vi "UHR-Fleezers Control (host) -Leonardo 04-2018 V2.vi"(0 "Tab Control":T5(tab)=enum."Trap Control (RF)") -> ()   [LabVIEW 2013] (continued)
  n83 = local write "Ave. Period (s)"(w194) -> ()
  n84 = property on="2D or 1D Scan" class="Bool (strict)"("Val(Sgnl)"=w149) -> ()  [unwired: 2 in, 2 out]
  n85 = xnode "Read/Write Control"("FPGA VI Reference In"=w146, "error in"=w165, "ai count"="AI Count (ticks)", "Interlace ON/OFF"=w132, "Number Interlace Cycles"=w131, "Set 1"=w12, "Set 2"=w11, "Set 3"=w10, "FB On/Off Set 1"=w252, "FB On/Off Set 2"=w251, "Interlace Off Parameters"=w130, "FB Setpoint Set 1"=w243, "FB Setpoint Set 2"=w242, "FB Gains"="PID gains", "FB output range"=cluster{"output high":i16, "output low":i16} {"output high"=3000, "output low"=0} ("FB output range 1"), "Cycles per step"=w228, "Scan BD"=w240, "Number of scans"=w224, "Scan steps"=w229, "Scan freq.  increment"=w230, "AO1 (Y)"=w212, "AO2 (X)"=w211, "Scan freq.  increment (MCL)"=w205, "Scan steps (MCL)"=w204, "Cycles per step (MCL)"=w203, "Number of scans (MCL)"=w202, "MCL count"=w129, "Cont. Scan (MCL)"=w201, "MCL Scan Axis"=w195, "1D or 2D Scan?"=w149, "N of AI1 Int Acq Sets"=w185, "BD 1 Delay (ticks)"="Freq switch delay", "Amp switch delay"="Amp switch delay", "Swap F1 and F2"="Swap F1 and F2", "APD Acq Rate Count"=w154, "APD to FIFO"=FALSE, "APD Gate Operating Mode"="APD Gate", "APD Gate ON Count"="APD Gate ON Count", "APD Gate OFF Count"="APD Gate OFF Count", "Invert APD Gate"="Invert APD Gate", "DIO count 1 (ticks)"="DIO count 1 (ticks)", "DIO count 2 (ticks)"="DIO count 2 (ticks)", "DIO count 3 (ticks)"="DIO count 3 (ticks)", "APD 1 AO scale factor"="APD 1 AO Mult.", "APD 2 AO scale factor"="APD 2 AO Mult.", "Diff FB Measurement?"=w17, "Dynamic Force FB (Ronen)"=w16, "Negate Diff?"=w15, "Next trap write delay (ticks)"="Next trap write delay (ticks)", "Phase offset method"="Phase offset method", "Phase Trap 1"="Phase increment trap 1", "RF phase reset before cycles"="RF phase reset before cycles", "Phase Trap 2"="Phase increment trap 2") -> ("FPGA VI Reference Out"=w124:T20, "error out"=w126:errorcluster)  [unwired: 1 in]
  n86 = local read "Green Laser ON/Interlacing"() -> (w127:bool)
  n87 = local read "Green laser mode"() -> (w128:enum32{"Laser ON", "Laser OFF", "Interlace"})
  n88 = local read "GI Frequency, OFF count"() -> (w120:u32)
  n89 = local read "GI Frequency, ON count"() -> (w119:u32)
  n90 = Multiply(x="Current When FB OFF (%)", y=655.35) -> (x*y=w110:dbl)
  n91 = local read "Green FB Count"() -> (w118:u32)
  n92 = Multiply(x="Green FB Setpoint (mV)", y=3.2767) -> (x*y=w107:dbl)
  n93 = To Unsigned Word Integer(number=w110) -> (unsigned 16bit integer=w108:u16)
  n94 = local read "Invert GI"() -> (w122:bool)
  n95 = To Word Integer(number=w107) -> (16bit integer=w105:i16)
  n96 = case shown="True" w127 {
    tunnel: w128 -> [_ w287]
    tunnel: [enum32{"Laser ON", "Laser OFF", "Interlace"}."Laser OFF" ("Green laser mode") w287] -> w121
    frame False {
    }
    frame True {
    }
  }
  n97 = local read "Trap Pos. AI1 X Pre-scale"() -> (w78:u16)
  n98 = local read "Trap Pos FB Monitor\nT1 or T2"() -> (w85:bool)
  n99 = local read "Trap Pos FB Int Count"() -> (w73:u16)
  n100 = local read "Trap Pos FB Negate Action"() -> (w84:bool)
  n101 = local read "Trap Pos. FB Offset Factor"() -> (w83:i64)
  n102 = local read "Trap Pos. FB Mult Factor"() -> (w82:i64)
  n103 = local read "Trap Pos. FB Gains"() -> (w80:T11)
  n104 = local read "Trap Pos. FB Range"() -> (w81:T12)
  n105 = xnode "Read/Write Control"("FPGA VI Reference In"=w124, "error in"=w126, "Green interlace ON count 2"=w119, "Green interlace OFF count 2"=w120, "Invert GI 2"=w122, "Operating Mode 2"=w121, "Green FB Gains"="Green FB Gains", "Green FB Setpoint"=w105, "Green FB On/Off"="Green FB On/Off", "Current Out"=w108, "Green int current ON count adj"="Green int current ON count adj", "Green FB Count"=w118, "Operating Mode"=w121, "Green interlace OFF count"=w120, "Green interlace ON count"=w119, "Invert GI"=w122, "Trap Pos FB Monitor T1 or T2"=w85, "Trap Pos FB Negate Action"=w84, "Trap Pos. FB Offset Factor"=w83, "Trap Pos. FB Mult Factor"=w82, "Trap pos. FB Range"=w81, "Trap Pos. FB Gains"=w80, "Force feedback"=FALSE, "AI1 X Scale"=w78, "Trap Pos to FIFO"=TRUE, "Trap Pos FB Int Count"=w73) -> ("FPGA VI Reference Out"=w123:T20, "error out"=w125:errorcluster)
  n106 = xnode "Invoke Method"("FPGA VI Reference In"=w123, "error in"=w125, "Requested Depth"="Trap AI FIFO Depth") -> ("FPGA VI Reference Out"=w88:T20, "error out"=w87:errorcluster)  [unwired: 1 out]
  n107 = xnode "Invoke Method"("FPGA VI Reference In"=w88, "error in"=w87, "Requested Depth"="Trap Position FIFO Depth") -> ("FPGA VI Reference Out"=w75:T20, "error out"=w74:errorcluster)  [unwired: 1 out]
  n108 = flat-sequence {
    tunnel: w147 -> [w292]
    tunnel: [w292] -> w146
    tunnel: [w291] -> w33
    tunnel: [w290] -> w145
    tunnel: [w288] -> w143
    tunnel: [w289] -> w144
    frame #0 {
      w289 = T16 {"Minimum"=60.0, "Maximum"=90.0, "Increment"=1.0} ("Min Max Inc")
      w288 = T16 {"Minimum"=0.0, "Maximum"=75.0, "Increment"=1.0} ("Data Entry Limits")
      w291 = T16 {"Minimum"=60.0, "Maximum"=90.0, "Increment"=1.0} ("Min Max Inc")
      w290 = T16 {"Minimum"=0.0, "Maximum"=75.0, "Increment"=1.0} ("Data Entry Limits")
      n109 = property on="BD 2 Frequency 1 (MHz)" class="DigNum (strict)"("Data Range"=w289) -> ()  [unwired: 2 in, 2 out]
      n110 = property on="BD 2 Frequency 3 (MHz)" class="DigNum (strict)"("Data Range"=w289) -> ()  [unwired: 2 in, 2 out]
      n111 = property on="BD 2 Frequency 2 (MHz)" class="DigNum (strict)"("Data Range"=w289) -> ()  [unwired: 2 in, 2 out]
      n112 = property on="BD 1 Frequency 1 (MHz)" class="DigNum (strict)"("Data Range"=w291) -> ()  [unwired: 2 in, 2 out]
      n113 = property on="BD 1 Frequency 2 (MHz)" class="DigNum (strict)"("Data Range"=w291) -> ()  [unwired: 2 in, 2 out]
      n114 = property on="BD 1 Frequency 3 (MHz)" class="DigNum (strict)"("Data Range"=w291) -> ()  [unwired: 2 in, 2 out]
      n115 = property on="BD 2 Amplitude 1 (%)" class="DigNum (strict)"("Data Range"=w288) -> ()  [unwired: 2 in, 2 out]
      n116 = property on="BD 2 Amplitude 2 (%)" class="DigNum (strict)"("Data Range"=w288) -> ()  [unwired: 2 in, 2 out]
      n117 = property on="BD 2 Amplitude 3 (%)" class="DigNum (strict)"("Data Range"=w288) -> ()  [unwired: 2 in, 2 out]
      n118 = property on="BD 1 Amplitude 3 (%)" class="DigNum (strict)"("Data Range"=w290) -> ()  [unwired: 2 in, 2 out]
      n119 = property on="BD 1 Amplitude 2 (%)" class="DigNum (strict)"("Data Range"=w290) -> ()  [unwired: 2 in, 2 out]
      n120 = property on="BD 1 Amplitude 1 (%)" class="DigNum (strict)"("Data Range"=w290) -> ()  [unwired: 2 in, 2 out]
      "X RF Frequency Limits (MHz)" <- w291
      "X RF Amplitude Limits (%)" <- w290
      "Y RF Amplitude Limits (%)" <- w288
      "Y RF Frequency Limits (MHz)" <- w289
    }
  }
  n121 = xnode "Invoke Method"("FPGA VI Reference In"=w75, "error in"=w74) -> ("FPGA VI Reference Out"=w53:T20, "error out"=w52:errorcluster)  [unwired: 1 in]
  n122 = flat-sequence "Initial FPGA Loop Relative Phase Adjustment" {
    tunnel: "Initial Phase Adjustment (GI) 2" -> [w294]
    tunnel: "Initial Phase Adj. (MCL)" -> [w295]
    tunnel: w52 -> [w296]
    tunnel: w53 -> [w297]
    tunnel: "Initial Phase Adjustment (GI)" -> [w298]
    tunnel: "Initial Phase Adjustment (AI1)" -> [w299]
    tunnel: [w299] -> w61
    tunnel: [w298] -> w60
    tunnel: [w297] -> w59
    tunnel: [w296] -> w58
    tunnel: [w295] -> w57
    tunnel: [w294] -> w56
    tunnel: [w310] -> w171
    tunnel: [w304] -> w169
    tunnel: "Initial Phase Adjustment (APD Acq)" -> [w303]
    tunnel: "Initial Phase Adjustment (APD 1 Gate)" -> [w302]
    tunnel: "Initial Phase Adjustment (Green FB)" -> [w301]
    tunnel: w61 -> [w309]
    tunnel: w60 -> [w308]
    tunnel: w59 -> [w307]
    tunnel: w58 -> [w306]
    tunnel: w57 -> [w305]
    tunnel: w56 -> [w300]
    tunnel: w171 -> [w312]
    tunnel: [w313] -> w170
    tunnel: w169 -> [w313]
    tunnel: [w312] -> w168
    tunnel: w170 -> [w316]
    tunnel: w168 -> [w315]
    tunnel: [w318] -> w167
    tunnel: [w317] -> w166
    tunnel: [w320] -> w51
    tunnel: [w321] -> w54
    tunnel: w167 -> [w321]
    tunnel: w166 -> [w320]
    frame #0 {
      n123 = Wait (ms)(milliseconds to wait=u32 1000) -> ()  [unwired: 1 out]
    }
    frame #1 {
      n124 = xnode "Read/Write Control"("FPGA VI Reference In"=w307, "error in"=w306, "Phase count adjustment"=w309, "Phase count adjustment (GI)"=w308, "Phase count adjustment (MCL)"=w305, "Phase Count Adjustment (APD Acq)"=w303, "Phase count adjustment (APD 1 Gate)"=w302, "Phase count adjustment (Green FB)"=w301, "Phase count adjustment (GI) 2"=w300) -> ("FPGA VI Reference Out"=w304:T20, "error out"=w310:errorcluster)
    }
    frame #2 {
      n125 = Wait (ms)(milliseconds to wait=u32 1000) -> ()  [unwired: 1 out]
    }
    frame #3 {
      w314 = TRUE
      n126 = xnode "Read/Write Control"("FPGA VI Reference In"=w316, "error in"=w315, "+ phase"=w314, "+ phase (GI)"=w314, "+ phase (MCL)"=w314, "+ phase (APD Acq)"=w314, "+ phase (APD 1 Gate)"=w314, "+ phase (Green FB)"=w314, "+ phase (GI) 2"=w314) -> ("FPGA VI Reference Out"=w317:T20, "error out"=w318:errorcluster)
    }
    frame #4 {
      n127 = Wait (ms)(milliseconds to wait=u32 1000) -> ()  [unwired: 1 out]
    }
  }
  n128 = Unbundle By Name(w33) -> ("Minimum"=w32:dbl, "Maximum"=w31:dbl)
  n129 = local read "Phase adj. (Green FB)"() -> (w141:i16)
  n130 = local read "Phase adj. (GI) 2"() -> (w111:i16)
  n131 = local read "Phase adjust (MCL)"() -> (w196:i16)
  n132 = local read "Phase adj. (AI1)"() -> (w198:i16)
  n133 = local read "Phase adj. (GI)"() -> (w197:i16)
  n134 = Multiply(x=w32, y=w30) -> (x*y=w28:dbl)
  n135 = Multiply(x=w31, y=w30) -> (x*y=w29:dbl)
  n136 = Multiply(x=49152000.0, y=6.0) -> (x*y=w22:dbl)
  n137 = Scale By Power Of 2(n=w27, x=w28) -> (x*2^n=w24:dbl)
  n138 = Scale By Power Of 2(n=w27, x=w29) -> (x*2^n=w23:dbl)
  n139 = xnode "Read/Write Control"("FPGA VI Reference In"=w51, "error in"=w54, "Phase count adjustment"=w198, "Phase count adjustment (GI)"=w197, "Phase count adjustment (MCL)"=w196, "Phase Count Adjustment (APD Acq)"="Phase Adj. (APD Acq)", "Phase count adjustment (APD 1 Gate)"="Phase Adj. (APD 1 Gate)", "Phase count adjustment (Green FB)"=w141, "Phase count adjustment (GI) 2"=w111) -> ("FPGA VI Reference Out"=w8:T20, "error out"=w7:errorcluster)
  n140 = Divide(x=w23, y=w22) -> (x/y=w20:dbl)
  n141 = Divide(x=w24, y=w22) -> (x/y=w21:dbl)
  n142 = To Unsigned Quad Integer(1:w21) -> (0:w19:u64)
  n143 = To Unsigned Quad Integer(1:w20) -> (0:w18:u64)
  n144 = xnode "Read/Write Control"("FPGA VI Reference In"=w8, "FB Min frequency"=w19, "FB Max Frequency"=w18) -> ()  [unwired: 1 in, 2 out]
  n145 = call "set RF board frequency - interlace.vi"("Board 2 Frequency Limits"=w144, "Board 1 Frequency Limits"=w33, "error in"=w7, "FPGA VI Reference In"=w8, "Board 2 Frequency 3 (MHz)"="BD 2 Frequency 3 (MHz)", "Board 1 Frequency 3 (MHz)"="BD 1 Frequency 3 (MHz)", "Board 2 Frequency 2 (MHz)"="BD 2 Frequency 2 (MHz)", "Board 2 Frequency 1 (MHz)"="BD 2 Frequency 1 (MHz)", "Board 1 Frequency 2 (MHz)"="BD 1 Frequency 2 (MHz)", "Board 1 Frequency 1  (MHz)"="BD 1 Frequency 1 (MHz)") -> ("error out"=w263:errorcluster, "FPGA VI Reference Out"=w264:T20)
  n146 = call "set RF board amplitude - interlace.vi"("Board 2 Amplitude Limits"=w143, "Board 1 Amplitude Limits"=w145, "error in"=w263, "FPGA VI Reference In"=w264, "Board 2 Amplitude 3 (%)"="BD 2 Amplitude 3 (%)", "Board 1 Amplitude 3 (%)"="BD 1 Amplitude 3 (%)", "Board 2 Amplitude 2 (%)"="BD 2 Amplitude 2 (%)", "Board 2 Amplitude 1 (%)"="BD 2 Amplitude 1 (%)", "Board 1 Amplitude 2 (%)"="BD 1 Amplitude 2 (%)", "Board 1 Amplitude 1 (%)"="BD 1 Amplitude 1 (%)") -> ("error out"=w49:errorcluster, "FPGA VI Reference Out"=w50:T20)
  n147 = flat-sequence {
    tunnel: w50 -> [w323]
    tunnel: w49 -> [w322]
    tunnel: [w323] -> w256
    tunnel: [w322] -> w255
    tunnel: [w331] -> w254
    tunnel: w256 -> [w331]
    tunnel: [w330] -> w253
    tunnel: w255 -> [w330]
    tunnel: w254 -> [w334]
    tunnel: w253 -> [w333]
    tunnel: [w334] -> w45
    tunnel: [w333] -> w44
    tunnel: [w340] -> w70
    tunnel: [w344] -> w55
    tunnel: w45 -> [w344]
    tunnel: w44 -> [w339]
    frame #0 {
      n148 = local read "Trap 1 (ON/OFF)"() -> (w324:bool)
      n149 = local write "Saving..."(FALSE ("Saving Data")) -> ()
      n150 = local write "Stop All"(FALSE ("Stop All")) -> ()
      n151 = local write "Index"(1.0 ("Index")) -> ()
      n152 = property on="Trap 1 ON" class="Bool (strict)"("Value"=w324) -> ()  [unwired: 2 in, 2 out]
      "Manipulating Trap" <- FALSE ("Manipulating Trap")
    }
    frame #1 {
      n153 = local read "Trap 2 (ON/OFF)"() -> (w329:bool)
      n154 = Wait (ms)(milliseconds to wait=u32 50) -> ()  [unwired: 1 out]
      n155 = property on="Trap 2 ON" class="Bool (strict)"("Val(Sgnl)"=w329) -> ()  [unwired: 2 in, 2 out]
    }
    frame #2 {
      n156 = local read "Scan Range (nm)"() -> (w335:dbl)
      n157 = call "Update messages.vi"("Message to add"="UHR-Fleezers ready.", "Old message string"="") -> ("New message string"=w338:string)
      n158 = local write "Messages"(w338) -> ()
      n159 = property on="Scan Range (nm)" class="DigNum (strict)"("Val(Sgnl)"=w335) -> ()  [unwired: 2 in, 2 out]
    }
    frame #3 {
      n160 = call "hamilton_controller.vi"("error in"=w339, "action"=T21."CONNECT") -> ("error out"=w341:errorcluster)  [unwired: 9 in]
      n161 = call "hamilton_controller.vi"("error in"=w341, "action"=T21."INITIALIZE VALVES") -> ("error out"=w340:errorcluster)  [unwired: 9 in]
    }
  }
  n162 = Subtract(x="BD 1 Frequency 1 (MHz)", y="BD 1 Frequency 2 (MHz)") -> (x-y=w184:dbl)
  n163 = Subtract(x="BD 2 Frequency 1 (MHz)", y="BD 2 Frequency 2 (MHz)") -> (x-y=w183:dbl)
  n164 = Square(x=w183) -> (x^2=w181:dbl)
  n165 = Square(x=w184) -> (x^2=w182:dbl)
  n166 = Add(x=w182, y=w181) -> (x+y=w180:dbl)
  n167 = Square Root(x=w180) -> (sqrt(x)=w179:dbl)
  n168 = local write "Trap Delta (MHz)"(w179) -> ()
  n169 = call "IMAQ Create"("Image Name"="APD 1 Image", "Image Type"=w94) -> ("New Image"=w93:T3)  [unwired: 3 in, 1 out]
  n170 = call "IMAQ Create"("Image Name"="APD 2 Image", "Image Type"=w94) -> ("New Image"=w92:T3)  [unwired: 3 in, 1 out]
  n171 = call "IMAQ Create"("Image Name"="Det. X Image", "Image Type"=w94) -> ("New Image"=w91:T3)  [unwired: 3 in, 1 out]
  n172 = call "IMAQ Create"("Image Name"="Det. Y Image", "Image Type"=w94) -> ("New Image"=w90:T3)  [unwired: 3 in, 1 out]
  n173 = Bundle("New Image"=w93, "New Image"=w92, "New Image"=w91, "New Image"=w90) -> (w89:T22)  [unwired: 1 in]
  n174 = Current VI's Path() -> (path=w34:path)
  n175 = Concatenate Strings("N.D.", "\r\n") -> (w38:string)
  n176 = Strip Path(path=w34) -> (stripped path=w35:path)  [unwired: 1 out]
  n177 = Initialize Array(w38, 4, 3) -> (w41:string[][])
  n178 = Build Path(base path=w35, name or relative path="Locations.txt") -> (appended path=→"Location path":path)
  n179 = local write "Location Matrix"(w41) -> ()
  n180 = while {
    stop <- w345 stop-if-true
    n181 = event shown="[0] Timeout" {
      selector: _ -> [_ _ _ _ _ _ _ _]
      dyn-events: _ -> [_ _ _ _ _ _ _ _]
      timeout: 10 -> [_ _ _ _ _ _ _ _]
      tunnel: [FALSE _ _ _ _ _ _ TRUE] -> w345
      event Timeout {
        # "Change the trajectory mode to Jog"
        # "Query and display stage positions"
        # "Setting ESP300 left and right limits for Z-axis, input in mm"
        # "Display Selected Location"
        n182 = event-data() -> ()  [unwired: 1 in, 2 out]
        n183 = local read "Capture Locations"() -> (w370:i32)
        n184 = local read "Location Matrix"() -> (w371:string[][])
        n185 = Concatenate Strings("1TP;\n2TP;\n3TP;\n1MD?;\n2MD?;\n3MD?" ("Substring"), "\r") -> (w354:string)
        n186 = local read "ESP Port"() -> (w357:refnum<visa-resource-name>)
        n187 = Index Array(array=w371, index (row)=w370) -> (element=w369:string[])  [unwired: 1 in]
        n188 = local read "ESP Port"() -> (w366:refnum<visa-resource-name>)
        n189 = VISA Write(VISA resource name=w357, write buffer=w354, error in (no error)="error in") -> (VISA resource name out=w355:refnum<visa-resource-name>, error out=w353:errorcluster)  [unwired: 1 out]
        n190 = Concatenate Strings("3SL" ("Substring"), "ESP ZL-Limit", ";3SR", "ESP ZR-Limit", "\r") -> (w365:string)
        n191 = Array To Cluster(array=w369) -> (cluster=w368:T23)
        n192 = case shown="True" TRUE ("Case Constant\n(See Context Help)") {
          tunnel: w355 -> [_ w409]
          tunnel: w353 -> [w390 w408]
          tunnel: [w390 w392] -> w359
          frame False {
          }
          frame True {
            w402 = u16 10 items=["1.0"=10, "1.5"=15, "2.0"=20] ("Serial Settings:Stop Bits")
            w403 = u16 0 items=["None", "Odd", "Even", "Mark", "Space"] ("Serial Settings:Parity")
            n193 = property class="Instr"(reference=w409, error in=w408, "Baud"=u32 921600 ("Serial Settings:Baud Rate"), "Data Bits"=u16 8 ("Serial Settings:Data Bits"), "Parity"=w403, "Stop Bits"=w402) -> (reference out=w407:refnum<visa-resource-name>, error out=w406:errorcluster, "Bytes at Port"=w391:u32)
            n194 = Wait (ms)(milliseconds to wait=u32 10) -> ()  [unwired: 1 out]
            n195 = VISA Read(VISA resource name=w407, byte count=w391, error in (no error)=w406) -> (VISA resource name out=w415:refnum<visa-resource-name>, read buffer=→"X Pos":string, error out=w416:errorcluster)  [unwired: 1 out]
            n196 = VISA Read(VISA resource name=w415, byte count=w391, error in (no error)=w416) -> (VISA resource name out=w413:refnum<visa-resource-name>, read buffer=→"Y Pos":string, error out=w414:errorcluster)  [unwired: 1 out]
            n197 = VISA Read(VISA resource name=w413, byte count=w391, error in (no error)=w414) -> (VISA resource name out=w401:refnum<visa-resource-name>, read buffer=→"Z Pos Pos":string, error out=w400:errorcluster)  [unwired: 1 out]
            n198 = VISA Read(VISA resource name=w401, byte count=w391, error in (no error)=w400) -> (VISA resource name out=w397:refnum<visa-resource-name>, read buffer=→"X Motion":string, error out=w398:errorcluster)  [unwired: 1 out]
            n199 = VISA Read(VISA resource name=w397, byte count=w391, error in (no error)=w398) -> (VISA resource name out=w396:refnum<visa-resource-name>, read buffer=→"Y Motion":string, error out=w394:errorcluster)  [unwired: 1 out]
            n200 = VISA Read(VISA resource name=w396, byte count=w391, error in (no error)=w394) -> (read buffer=→"Z motion":string, error out=w392:errorcluster)  [unwired: 2 out]
          }
        }
        "error out" <- w359
        n201 = VISA Write(VISA resource name=w366, write buffer=w365) -> ()  [unwired: 1 in, 3 out]
        n202 = local write item#477(w368) -> ()
        n203 = disable-structure shown="Disabled" {
          frame Disabled {
            # "Change Low Jog Velocity"
            # "Change High Jog Velocity"
            n204 = Concatenate Strings("1JH" ("Substring"), "Axis 1", "2JH" ("Substring"), "Axis 2", "3JH" ("Substring"), "Axis 3", "\r") -> (w389:string)
            n205 = local read "ESP Port"() -> (w388:refnum<visa-resource-name>)
            n206 = VISA Write(VISA resource name=w388, write buffer=w389) -> ()  [unwired: 1 in, 3 out]
            n207 = Concatenate Strings("1JW" ("Substring"), "Axis 1", "2JW" ("Substring"), "Axis 2", "3JW" ("Substring"), "Axis 3", "\r") -> (w380:string)
            n208 = local read "ESP Port"() -> (w379:refnum<visa-resource-name>)
            n209 = VISA Write(VISA resource name=w379, write buffer=w380) -> ()  [unwired: 1 in, 3 out]
          }
          frame Enabled {
          }
        }
        n210 = local read "ESP Port"() -> (w347:refnum<visa-resource-name>)
        n211 = Concatenate Strings("1TJ3;\n2TJ3;\n3TJ3" ("Substring"), "\r") -> (w348:string)
        n212 = VISA Write(VISA resource name=w347, write buffer=w348) -> ()  [unwired: 1 in, 3 out]
      }
      event "Goto Top (F6)": Value Change {
        n213 = event-data() -> ()  [unwired: 1 in, 5 out]
        n214 = stacked-sequence {
          frame #0 {
            # "stop motions of all axes before going to avoid reversing of direction"
            n215 = local read "ESP Port"() -> (w421:refnum<visa-resource-name>)
            n216 = Concatenate Strings("ST" ("Substring"), "\r") -> (w418:string)
            n217 = VISA Write(VISA resource name=w421, write buffer=w418) -> ()  [unwired: 1 in, 3 out]
          }
          frame #1 {
            n218 = Wait (ms)(milliseconds to wait=u32 50) -> ()  [unwired: 1 out]
          }
          frame #2 {
            # "Change the trajectory mode to Trapezoidal"
            n219 = local read "ESP Port"() -> (w426:refnum<visa-resource-name>)
            n220 = Concatenate Strings("1TJ1;\n2TJ1;\n3TJ1" ("Substring"), "\r") -> (w423:string)
            n221 = VISA Write(VISA resource name=w426, write buffer=w423) -> ()  [unwired: 1 in, 3 out]
          }
          frame #3 {
            # "Go to Top Dispensor"
            n222 = local read "Location Matrix"() -> (w438:string[][])
            n223 = Index Array(array=w438, index (row)=0) -> (element=w434:string[])  [unwired: 1 in]
            n224 = Decimate 1D Array(w434) -> (w432:string[], w430:string[], w428:string[])
            n225 = local read "ESP Port"() -> (w435:refnum<visa-resource-name>)
            n226 = Concatenate Strings("1PA" ("Substring"), w432, "2PA" ("Substring"), w430, "3PA" ("Substring"), w428, "\r") -> (w436:string)
            n227 = VISA Write(VISA resource name=w435, write buffer=w436) -> ()  [unwired: 1 in, 3 out]
          }
          frame #4 {
            n228 = Wait (ms)(milliseconds to wait=u32 100) -> ()  [unwired: 1 out]
          }
          frame #5 {
            # "Change the trajectory mode to Jog"
            n229 = local read "ESP Port"() -> (w443:refnum<visa-resource-name>)
            n230 = Concatenate Strings("1TJ3;\n2TJ3;\n3TJ3" ("Substring"), "\r") -> (w440:string)
            n231 = VISA Write(VISA resource name=w443, write buffer=w440) -> ()  [unwired: 1 in, 3 out]
          }
        }
      }
      event "Goto Exp (F8)": Value Change {
        n232 = event-data() -> ()  [unwired: 1 in, 5 out]
        n233 = stacked-sequence {
          frame #0 {
            # "stop motions of all axes before going to avoid reversing of direction"
            n234 = local read "ESP Port"() -> (w447:refnum<visa-resource-name>)
            n235 = Concatenate Strings("ST" ("Substring"), "\r") -> (w444:string)
            n236 = VISA Write(VISA resource name=w447, write buffer=w444) -> ()  [unwired: 1 in, 3 out]
          }
          frame #1 {
            n237 = Wait (ms)(milliseconds to wait=u32 50) -> ()  [unwired: 1 out]
          }
          frame #2 {
            # "Change the trajectory mode to Trapezoidal"
            n238 = local read "ESP Port"() -> (w452:refnum<visa-resource-name>)
            n239 = Concatenate Strings("1TJ1;\n2TJ1;\n3TJ1" ("Substring"), "\r") -> (w449:string)
            n240 = VISA Write(VISA resource name=w452, write buffer=w449) -> ()  [unwired: 1 in, 3 out]
          }
          frame #3 {
            # "Go to Experimental"
            n241 = local read "Location Matrix"() -> (w464:string[][])
            n242 = Index Array(array=w464, index (row)=2) -> (element=w460:string[])  [unwired: 1 in]
            n243 = Decimate 1D Array(w460) -> (w458:string[], w456:string[], w454:string[])
            n244 = Concatenate Strings("1PA" ("Substring"), w458, "2PA" ("Substring"), w456, "3PA" ("Substring"), w454, "\r") -> (w462:string)
            n245 = local read "ESP Port"() -> (w461:refnum<visa-resource-name>)
            n246 = VISA Write(VISA resource name=w461, write buffer=w462) -> ()  [unwired: 1 in, 3 out]
          }
          frame #4 {
            n247 = Wait (ms)(milliseconds to wait=u32 200) -> ()  [unwired: 1 out]
          }
          frame #5 {
            # "Change the trajectory mode to Jog"
            n248 = local read "ESP Port"() -> (w466:refnum<visa-resource-name>)
            n249 = Concatenate Strings("1TJ3;\n2TJ3;\n3TJ3" ("Substring"), "\r") -> (w469:string)
            n250 = VISA Write(VISA resource name=w466, write buffer=w469) -> ()  [unwired: 1 in, 3 out]
          }
        }
      }
      event "Goto Bottom (F7)": Value Change {
        n251 = event-data() -> ()  [unwired: 1 in, 5 out]
        n252 = stacked-sequence {
          frame #0 {
            # "stop motions of all axes before going to avoid reversing of direction"
            n253 = local read "ESP Port"() -> (w473:refnum<visa-resource-name>)
            n254 = Concatenate Strings("ST" ("Substring"), "\r") -> (w470:string)
            n255 = VISA Write(VISA resource name=w473, write buffer=w470) -> ()  [unwired: 1 in, 3 out]
          }
          frame #1 {
            n256 = Wait (ms)(milliseconds to wait=u32 50) -> ()  [unwired: 1 out]
          }
          frame #2 {
            # "Change the trajectory mode to Trapezoidal"
            n257 = local read "ESP Port"() -> (w478:refnum<visa-resource-name>)
            n258 = Concatenate Strings("1TJ1;\n2TJ1;\n3TJ1" ("Substring"), "\r") -> (w475:string)
            n259 = VISA Write(VISA resource name=w478, write buffer=w475) -> ()  [unwired: 1 in, 3 out]
          }
          frame #3 {
            # "Go to Bottom Dispensor"
            n260 = local read "Location Matrix"() -> (w490:string[][])
            n261 = Index Array(array=w490, index (row)=1) -> (element=w486:string[])  [unwired: 1 in]
            n262 = Decimate 1D Array(w486) -> (w484:string[], w482:string[], w480:string[])
            n263 = Concatenate Strings("1PA" ("Substring"), w484, "2PA" ("Substring"), w482, "3PA" ("Substring"), w480, "\r") -> (w488:string)
            n264 = local read "ESP Port"() -> (w487:refnum<visa-resource-name>)
            n265 = VISA Write(VISA resource name=w487, write buffer=w488) -> ()  [unwired: 1 in, 3 out]
          }
          frame #4 {
            n266 = Wait (ms)(milliseconds to wait=u32 200) -> ()  [unwired: 1 out]
          }
          frame #5 {
            # "Change the trajectory mode to Jog"
            n267 = local read "ESP Port"() -> (w492:refnum<visa-resource-name>)
            n268 = Concatenate Strings("1TJ3;\n2TJ3;\n3TJ3" ("Substring"), "\r") -> (w495:string)
            n269 = VISA Write(VISA resource name=w492, write buffer=w495) -> ()  [unwired: 1 in, 3 out]
          }
        }
      }
      event "Capture": Value Change {
        n270 = event-data() -> ()  [unwired: 1 in, 5 out]
        n271 = local read "Capture Locations"() -> (w496:i32)
        n272 = local read "Z Pos Pos"() -> (w497:string)
        n273 = local read "X Pos"() -> (w499:string)
        n274 = local read "Y Pos"() -> (w498:string)
        n275 = case shown="1" w496 {
          selector: w496 -> [w503 w510 w517 w524]
          tunnel: w499 -> [w506 w513 w520 w527]
          tunnel: w498 -> [w505 w512 w519 w526]
          tunnel: w497 -> [w504 w511 w518 w525]
          frame 0, Default {
            # "Capture Top Dispensor Location"
            n276 = local read "Location Matrix"() -> (w502:string[][])
            n277 = Build Array(w506, w505, w504) -> (w501:string[])
            n278 = Replace Array Subset(array=w502, new element=w501, index (row)=w503) -> (w500:string[][])  [unwired: 1 in]
            n279 = local write "Location Matrix"(w500) -> ()
          }
          frame 1 {
            # "Capture Bottom Dispensor Location"
            n280 = local read "Location Matrix"() -> (w509:string[][])
            n281 = Build Array(w513, w512, w511) -> (w508:string[])
            n282 = Replace Array Subset(array=w509, new element=w508, index (row)=w510) -> (w507:string[][])  [unwired: 1 in]
            n283 = local write "Location Matrix"(w507) -> ()
          }
          frame 2 {
            # "Capture Experimental Region Location"
            n284 = local read "Location Matrix"() -> (w516:string[][])
            n285 = Build Array(w520, w519, w518) -> (w515:string[])
            n286 = Replace Array Subset(array=w516, new element=w515, index (row)=w517) -> (w514:string[][])  [unwired: 1 in]
            n287 = local write "Location Matrix"(w514) -> ()
          }
          frame 3 {
            # "Capture Other Location"
            n288 = local read "Location Matrix"() -> (w523:string[][])
            n289 = Build Array(w527, w526, w525) -> (w522:string[])
            n290 = Replace Array Subset(array=w523, new element=w522, index (row)=w524) -> (w521:string[][])  [unwired: 1 in]
            n291 = local write "Location Matrix"(w521) -> ()
          }
        }
      }
      event "Save": Value Change {
        # "reshape Location Matrix to 1-D array to write"
        n292 = event-data() -> ()  [unwired: 1 in, 5 out]
        n293 = local read "Location Matrix"() -> (w531:string[][])
        n294 = local read "Location path"() -> (w528:path)
        n295 = Reshape Array(w531, 12) -> (w529:string[])
        n296 = Write to Text File(file (use dialog)=w528, text=w529) -> ()  [unwired: 2 in, 3 out]
      }
      event "Activate Joystick": Value Change {
        # "Change the trajectory mode to Jog"
        n297 = event-data() -> ()  [unwired: 1 in, 5 out]
        n298 = disable-structure shown="Disabled" {
          frame Disabled {
            n299 = case shown="True" "Activate Joystick" {
              frame False {
              }
              frame True {
                # "Change the trajectory mode to Jog"
                n300 = local read "ESP Port"() -> (w540:refnum<visa-resource-name>)
                n301 = Concatenate Strings("1TJ3;\n2TJ3;\n3TJ3" ("Substring"), "\r") -> (w537:string)
                n302 = VISA Write(VISA resource name=w540, write buffer=w537) -> ()  [unwired: 1 in, 3 out]
              }
            }
          }
          frame Enabled {
          }
        }
        n303 = local read "ESP Port"() -> (w532:refnum<visa-resource-name>)
        n304 = Concatenate Strings("1TJ3;\n2TJ3;\n3TJ3" ("Substring"), "\r") -> (w535:string)
        n305 = VISA Write(VISA resource name=w532, write buffer=w535) -> ()  [unwired: 1 in, 3 out]
      }
      event "Stop All": Mouse Down {
        n306 = event-data() -> ()  [unwired: 1 in, 5 out]
      }
    }
  }
  n307 = disable-structure shown="Disabled" {
    disable-tunnel: w55 -> [w570 _]
    frame Disabled {
      w565 = T17 0 items=["Grayscale (U8)", "Grayscale (I16)", "Grayscale (SGL)", "Complex (CSG)", "RGB (U32)", "HSL (U32)", "RGB (U64)", "Grayscale (U16)"] ("Image Type")
      n308 = call <vilib>:"IMAQ Init.vi"("Interface Name"="img0") -> ("error out"=w567:errorcluster, "IMAQ Session Out"=w569:refnum<k11>)  [unwired: 9 in]
      n309 = call <vilib>:"IMAQ Grab Setup.vi"("error in (no error)"=w567, "IMAQ Session In"=w569) -> ("error out"=w563:errorcluster, "IMAQ Session Out"=w564:refnum<k11>)  [unwired: 8 in]
      n310 = call "IMAQ Create"("Image Name"="untitled", "Image Type"=w565) -> ("New Image"=w562:T3)  [unwired: 3 in, 1 out]
      n311 = call <vilib>:"Application Directory.vi"() -> ("Application Directory"=w549:path)
      n312 = Build Path(base path=w549, name or relative path="_trap_screen_positions") -> (appended path=w557:path)
      n313 = Open/Create/Replace File(file path (use dialog)=w557, operation (0:open)=T24."open or create", access (0:read/write)=enum16{"read/write", "read-only", "write-only"}."read/write") -> (refnum out=w559:refnum<file>)  [unwired: 3 in, 2 out]
      n314 = local read "Trap Sets"() -> (w551:u32)
      n315 = for "Load trap positions on video screen from file." {
        N: w551 -> [_]
        tunnel: [w577] -> w552
        tunnel: w559 -> [w576]
        tunnel: [w573] -> w548 mode=indexing
        w575 = 4
        n316 = for {
          N: w575 -> [_]
          tunnel: [w581] -> w577
          tunnel: w576 -> [w580]
          tunnel: w575 -> [w579]
          tunnel: [w578] -> w574 mode=indexing
          n317 = Read from Binary File(5:w579, 11:w580) -> (2:w578:i32, 3:w581:refnum<file>)  [unwired: 4 in, 2 out]
        }
        n318 = Array To Cluster(array=w574) -> (cluster=w573:T28)
      }
      n319 = node-c288() -> (w572:T25)  [unwired: 4 in]
      n320 = timed-loop "acquire video and stage position" {
        timing: w572 -> [_]
        timing-out: [_] -> w571
        tunnel: w564 -> [w600]
        tunnel: w563 -> [w599]
        tunnel: w562 -> [w598]
        tunnel: [w597] -> w544
        tunnel: [w594] -> w545
        tunnel: [w595] -> w543
        tunnel: w570 -> [_]
        shift-right: [w591] -> w561
        shift-left: w548 -> [w592]
        tunnel: w551 -> [w589]
        stop <- w596 stop-if-true
        n321 = node-c288() -> ()  [unwired: 1 in, 1 out]
        n322 = event shown="[0] Timeout" {
          selector: _ -> [_ _ _ _]
          dyn-events: _ -> [_ _ _ _]
          timeout: 10 -> [_ _ _ _]
          tunnel: w600 -> [w611 w626 w635 w654]
          tunnel: w599 -> [w610 w628 w633 w656]
          tunnel: w598 -> [w609 w627 w634 w655]
          tunnel: [w608 w626 w635 w654] -> w597
          tunnel: [w601 w630 FALSE FALSE] -> w596
          tunnel: [w605 w628 w633 w656] -> w595
          tunnel: [w604 w627 w634 w655] -> w594
          tunnel: "radius" -> [_ _ w640 _]
          tunnel: w592 -> [w602 w629 w638 _]
          tunnel: [w602 w629 w639 cluster{i32, i32, i32, i32}[] []] -> w591
          tunnel: w589 -> [_ _ w631 _]
          event Timeout {
            n323 = event-data() -> ()  [unwired: 1 in, 2 out]
            n324 = call <vilib>:"IMAQ Grab Acquire.vi"("error in (no error)"=w610, "Image In"=w609, "IMAQ Session In"=w611) -> ("error out"=w606:errorcluster, "Image Out"=w607:T3, "IMAQ Session Out"=w608:refnum<k11>)  [unwired: 5 in, 1 out]
            n325 = case shown="True" "trap\nmarkers?" {
              tunnel: w602 -> [_ w619]
              tunnel: w607 -> [w613 w618]
              tunnel: w606 -> [w612 w617]
              tunnel: [w612 w616] -> w605
              tunnel: [w613 w614] -> w604
              frame False {
              }
              frame True {
                n326 = for {
                  tunnel: w619 -> [w625] mode=indexing
                  shift-right: [w623] -> w614
                  shift-left: w618 -> [w624]
                  tunnel: w617 -> [w622]
                  tunnel: [w621] -> w616
                  tunnel: u32 16711680 ("Color") -> [w620]
                  n327 = call "IMAQ Overlay Oval"("Color"=w620, "error in (no error)"=w622, "Bounding Rectangle"=w625, "Image"=w624) -> ("error out"=w621:errorcluster, "Image Out"=w623:T3)  [unwired: 6 in]
                }
              }
            }
            "Primary Video Display" <- w604
            n328 = Unbundle By Name(w606) -> ("status"=w601:bool)
          }
          event "Stop All": Value Change {
            n329 = event-data() -> ()  [unwired: 1 in, 5 out]
            n330 = local read "Stop All"() -> (w630:bool)
          }
          event "Primary Video Display": Mouse Down {
            n331 = event-data() -> ()  [unwired: 1 in, 7 out]
            n332 = Array Size(array=w638) -> (size(s)=w637:i32)
            n333 = Less?(x=w637, y=w631) -> (x < y?=w636:bool)
            n334 = case shown="True" w636 {
              tunnel: w640 -> [_ w650]
              tunnel: w638 -> [w641 w644]
              tunnel: [w641 w643] -> w639
              frame False {
              }
              frame True {
                n335 = property on="Primary Video Display" class="ImageControl"() -> ("Last Mouse Position"=w642:cluster{"X":i32, "Y":i32})  [unwired: 2 in, 2 out]
                n336 = Unbundle By Name(w642) -> ("X"=w652:i32, "Y"=w651:i32)
                n337 = Add(x=w651, y=w650) -> (x+y=w648:i32)
                n338 = Subtract(x=w651, y=w650) -> (x-y=w646:i32)
                n339 = Add(x=w652, y=w650) -> (x+y=w647:i32)
                n340 = Subtract(x=w652, y=w650) -> (x-y=w649:i32)
                n341 = Bundle(w649, w648, w647, w646) -> (w645:cluster{i32, i32, i32, i32})  [unwired: 1 in]
                n342 = Build Array (concatenate)(w644, w645) -> (w643:T29)
              }
            }
          }
          event "clear markers": Value Change {
            n343 = event-data() -> ()  [unwired: 1 in, 5 out]
          }
        }
        n344 = node-c288() -> ()  [unwired: 1 in, 1 out]
      }
      n345 = node-c288(w571) -> ()  [unwired: 1 out]
      n346 = Set File Position(offset (in bytes) (0)=i64 0, refnum=w552, from (0:start)=enum16{"start", "end", "current"}."start") -> (refnum out=w553:refnum<file>)  [unwired: 1 in, 1 out]
      n347 = for "Write trap positions to file so they can be remembered\nwhen program is removed from memory" {
        tunnel: w561 -> [w585] mode=indexing
        tunnel: [w583] -> w560
        tunnel: w553 -> [w582]
        n348 = Cluster To Array(cluster=w585) -> (array=w584:i32[])
        n349 = for {
          tunnel: w584 -> [w588] mode=indexing
          tunnel: [w587] -> w583
          tunnel: w582 -> [w586]
          n350 = Write to Binary File(file (use dialog)=w586, data=w588) -> (refnum out=w587:refnum<file>)  [unwired: 4 in, 2 out]
        }
      }
      n351 = Close File(refnum=w560) -> ()  [unwired: 1 in, 2 out]
      n352 = call "IMAQ Dispose"("Image"=w545, "error in (no error)"=w543) -> ("error out"=w542:errorcluster)  [unwired: 4 in]
      n353 = call <vilib>:"IMAQ Stop.vi"("error in (no error)"=w542, "IMAQ Session In"=w544) -> ("error out"=w546:errorcluster, "IMAQ Session Out"=w547:refnum<k11>)  [unwired: 8 in]
      n354 = call <vilib>:"IMAQ Close.vi"("error in (no error)"=w546, "IMAQ Session In"=w547) -> ()  [unwired: 9 in, 1 out]
    }
    frame Enabled {
    }
  }
  n355 = disable-structure shown="Enabled" {
    disable-tunnel: [w663 _] -> w65
    disable-tunnel: w55 -> [w662 _]
    frame Enabled {
      n356 = node-c288() -> (w665:T25)  [unwired: 4 out]
      n357 = timed-loop "Rough control of MCL mirror stage (debugging)" {
        tunnel: w662 -> [w668]
        tunnel: [w667] -> w663
        timing: w665 -> [_]
        timing-out: [_] -> w664
        stop <- w667 stop-if-true
        n358 = node-c288() -> ()  [unwired: 2 out]
        n359 = case shown="0, Default" "MCL Mode" {
          tunnel: w668 -> [_ w671 w718]
          frame 0, Default {
            # "manual positioning"
          }
          frame 1 {
            # "sinusoidal wave"
            n360 = node-c288() -> (w673:T25)  [unwired: 4 out]
            n361 = timed-loop "Oscillate MCL mirror" {
              timing: w673 -> [_]
              timing-out: [_] -> w672
              tunnel: w671 -> [w712]
              i -> [w711]
              stop <- w674 stop-if-true
              n362 = node-c288() -> (w710:i64)  [unwired: 1 out]
              n363 = Multiply(x="AO1", y=32767.0) -> (x*y=w706:dbl)
              n364 = Multiply(x="AO2", y=32767.0) -> (x*y=w701:dbl)
              n365 = Divide(x=w706, y=10.0) -> (x/y=w707:dbl)
              n366 = Divide(x=w701, y=10.0) -> (x/y=w702:dbl)
              n367 = To Word Integer(number=w707) -> (16bit integer=w699:i16)
              n368 = To Word Integer(number=w702) -> (16bit integer=w698:i16)
              n369 = Divide(x=w710, y=i64 1000) -> (x/y=w681:dbl)
              n370 = Multiply(x=w681, y=w711) -> (x*y=w692:dbl)
              n371 = Multiply(x="Osc. freq. (Hz) 2", y=6.283185307179586) -> (x*y=w693:dbl)
              n372 = Multiply(x=w693, y=w692) -> (x*y=w691:dbl)
              n373 = Sine(x=w691) -> (sin(x)=w690:dbl)
              n374 = Multiply(x=w690, y="Osc. amp. (V)") -> (x*y=w688:dbl)
              n375 = Add(x=w688, y="Osc. center (V)") -> (x+y=w686:dbl)
              n376 = Divide(x=w686, y=10.0) -> (x/y=w684:dbl)
              n377 = Multiply(x=w684, y=32767.0) -> (x*y=w679:dbl)
              n378 = Select(t=w679, s="Scan axis", f=w699) -> (s? t:f=w697:dbl)
              n379 = Select(t=w698, s="Scan axis", f=w679) -> (s? t:f=w696:dbl)
              n380 = local read "MCL Mode"() -> (w678:u16)
              n381 = Not Equal?(x=w678, y=u16 1) -> (x != y?=w675:bool)
              n382 = local read "Stop All"() -> (w676:bool)
              n383 = xnode "Read/Write Control"("FPGA VI Reference In"=w712, "AO1 (Y)"=w697, "AO2 (X)"=w696) -> ()  [unwired: 1 in, 2 out]
              n384 = Compound Arithmetic op=OR(w676, w675) -> (w674:bool)
              n385 = node-c288() -> ()  [unwired: 2 out]
            }
            n386 = node-c288(w672) -> ()  [unwired: 1 out]
          }
          frame 2 {
            # "linear scan"
            n387 = case shown="True" "Start Scan" {
              tunnel: w718 -> [_ w730]
              frame False {
              }
              frame True {
                n388 = Subtract(x="End (V)", y="Begin (V)") -> (x-y=w726:dbl)
                n389 = Decrement(x="N Points") -> (x-1=w725:dbl)
                n390 = Divide(x=w726, y=w725) -> (x/y=w723:dbl)
                n391 = for {
                  N: "N Points" -> [_]
                  tunnel: "Begin (V)" -> [w743]
                  tunnel: w730 -> [w735]
                  tunnel: [w734] -> w729 mode=indexing
                  tunnel: w723 -> [w733]
                  tunnel: [w731] -> w722 mode=indexing
                  i -> [w742]
                  n392 = Multiply(x=w733, y=w742) -> (x*y=w741:dbl)
                  n393 = Add(x=w743, y=w741) -> (x+y=w738:dbl)
                  n394 = local read "Scan axis"() -> (w732:bool)
                  n395 = local read "AO1"() -> (w740:dbl)
                  n396 = local read "AO2"() -> (w739:dbl)
                  n397 = Select(t=w738, s=w732, f=w740) -> (s? t:f=w737:dbl)
                  n398 = Select(t=w739, s=w732, f=w738) -> (s? t:f=w736:dbl)
                  n399 = flat-sequence {
                    tunnel: w737 -> [w747]
                    tunnel: w736 -> [w746]
                    tunnel: w735 -> [w744]
                    tunnel: [w757] -> w734
                    tunnel: [w756] -> w731
                    frame #0 {
                      w750 = 10.0 ("y")
                      w745 = 32767.0 ("y")
                      n400 = Multiply(x=w747, y=w745) -> (x*y=w753:dbl)
                      n401 = Multiply(x=w746, y=w745) -> (x*y=w751:dbl)
                      n402 = Divide(x=w753, y=w750) -> (x/y=w754:dbl)
                      n403 = Divide(x=w751, y=w750) -> (x/y=w752:dbl)
                      n404 = To Word Integer(number=w754) -> (16bit integer=w748:i16)
                      n405 = To Word Integer(number=w752) -> (16bit integer=w749:i16)
                      n406 = xnode "Read/Write Control"("FPGA VI Reference In"=w744, "AO1 (Y)"=w748, "AO2 (X)"=w749) -> ()  [unwired: 1 in, 2 out]
                    }
                    frame #1 {
                      n407 = Wait (ms)(milliseconds to wait="DAQ Delay (ms)") -> ()  [unwired: 1 out]
                    }
                    frame #2 {
                      n408 = local read "Slow mean"() -> (w757:dbl)
                      n409 = local read "Sigma"() -> (w756:dbl)
                    }
                  }
                }
                n410 = Bundle("Begin (V)"="Begin (V)", w723, w729) -> (→"MCL Scan":cluster{"Begin (V)":dbl, dbl, dbl[]})  [unwired: 1 out]
                n411 = Bundle("Begin (V)"="Begin (V)", w723, w722) -> (→"MCL Scan 2":cluster{"Begin (V)":dbl, dbl, dbl[]})  [unwired: 1 out]
              }
            }
          }
        }
        n412 = local read "Stop All"() -> (w667:bool)
        n413 = node-c288() -> ()  [unwired: 2 out]
      }
      n414 = node-c288(w664) -> ()  [unwired: 1 out]
    }
    frame Disabled {
    }
  }
  n415 = node-c288(2 ("Processor")) -> (w48:T25)  [unwired: 3 in]
  n416 = node-c288() -> (w97:T25)  [unwired: 4 in]
  n417 = timed-loop "Control parameters (event loop)" {
    tunnel: w55 -> [w763]
    shift-right: [w762] -> _
    shift-left: errorcluster {"status"=FALSE, "code"=0, "source"=""} ("error out") -> [w761]
    tunnel: [w760] -> w67
    timing: w48 -> [_]
    timing-out: [_] -> w47
    stop <- w760 stop-if-true
    n418 = node-c288() -> ()  [unwired: 1 in, 1 out]
    n419 = event shown="[23] \"Phase Adj. (APD Acq)\", \"+ phase (APD Acq)\", \"- phase (APD Acq)\": Value Change" {
      selector: _ -> [_ _ _ _ _ _ _ _ _ _ _ _ _ _ _ _ _ _ _ _ _ _ _ _ _ _ _ _ _ _ _ _ _ _ _ _ _ _ _ _ _ _ _ _ _ _ _ _ _ _ _ _ _ _ _ _ _ _ _]
      dyn-events: _ -> [_ _ _ _ _ _ _ _ _ _ _ _ _ _ _ _ _ _ _ _ _ _ _ _ _ _ _ _ _ _ _ _ _ _ _ _ _ _ _ _ _ _ _ _ _ _ _ _ _ _ _ _ _ _ _ _ _ _ _]
      timeout: _ -> [_ _ _ _ _ _ _ _ _ _ _ _ _ _ _ _ _ _ _ _ _ _ _ _ _ _ _ _ _ _ _ _ _ _ _ _ _ _ _ _ _ _ _ _ _ _ _ _ _ _ _ _ _ _ _ _ _ _ _]
      tunnel: w763 -> [w804 _ _ _ w841 _ w859 w865 _ _ _ _ w942 _ _ w986 w992 w996 w1001 w1037 w1055 w1062 w1080 w1091 w1102 w1113 w1124 w1142 w1148 w1242 _ w1254 w1292 _ w1352 w1356 w1367 w1372 w1396 _ w1404 _ _ _ _ _ w1540 _ w1557 w1572 w1598 w1601 w1602 w1662 _ w1679 w1681 _ _]
      tunnel: [w803 _ _ _ w831 _ _ w864 _ _ w907 _ w922 _ _ w985 w988 w995 w998 w1036 w1053 w1061 w1074 w1085 w1096 w1107 w1118 w1140 w1147 w1240 _ w1252 w1290 _ w1350 w1354 w1357 w1370 w1394 _ w1402 _ _ _ _ _ w1538 _ _ _ _ _ _ _ _ _ _ _ _] -> w762
      tunnel: w761 -> [w802 _ _ _ w840 _ _ w863 _ _ w907 _ w941 _ _ w984 w987 w994 w997 w1035 w1054 w1060 w1079 w1090 w1101 w1112 w1123 w1141 w1146 w1241 _ w1253 w1291 _ w1351 w1355 w1366 w1371 w1395 _ w1403 _ _ _ _ _ w1539 _ w1556 w1571 w1597 w1600 w1603 w1661 _ w1678 _ _ _]
      tunnel: [_ _ _ _ _ _ _ _ _ _ w906 _ _ _ _ _ _ _ _ _ _ _ _ _ _ _ _ _ _ _ _ _ _ _ _ _ _ _ _ _ _ _ _ _ _ _ _ _ _ _ _ _ _ _ _ _ _ _ _] -> w760
      tunnel: [_ _ _ _ _ _ _ _ "Round T1 X" _ _ _ _ _ _ _ _ _ _ _ _ _ _ _ _ _ _ _ _ _ _ _ _ _ _ _ _ _ _ _ _ _ _ _ _ _ _ _ _ _ _ _ _ _ _ _ _ _ _] -> _
      tunnel: [_ _ _ "Adjust Scale\nto Mean" _ _ _ _ _ _ _ _ _ _ _ _ _ _ _ _ _ _ _ _ _ _ _ _ _ _ _ _ _ _ _ _ _ _ _ _ _ _ _ _ _ _ _ _ _ _ _ _ _ "Set SP to Reading" _ _ _ _ _] -> _
      tunnel: [_ _ _ _ _ _ _ _ _ "Round T2 X" _ "Delayed Interlace Start" _ _ _ _ _ _ _ _ _ _ _ _ _ _ _ _ _ _ _ _ _ _ _ _ _ _ _ _ _ _ _ _ _ _ _ _ _ _ _ _ _ _ _ _ _ _ _] -> _
      event "AI Count (ticks)", "Sets to FIFO (Traps)", "Save ave N", "FPGA Ave.", "# Samples/channel", "N sets to save": Value Change {
        # "So that if 'Save ave N' is updated, the AOD scanning code updates too."
        n420 = event-data() -> ()  [unwired: 6 out]
        n421 = local read "AI Count (ticks)"() -> (w785:u32)
        n422 = Unbundle By Name("Sets to FIFO (Traps)") -> ("Set 1"=w768:bool, "Set 2"=w767:bool, "Set 3"=w766:bool)
        n423 = Boolean To (0,1)(Boolean="Sets to FIFO (Traps)") -> (0, 1=w794:cluster{"Set 1":i16, "Set 2":i16, "Set 3":i16})
        n424 = xnode "Read/Write Control"("FPGA VI Reference In"=w804, "error in"=w802, "ai count"=w785, "Set 1"=w768, "Set 2"=w767, "Set 3"=w766, "N of AI1 Int Acq Sets"="N Acq Sets (Traps + Fl.)") -> ("error out"=w803:errorcluster)  [unwired: 1 out]
        n425 = Cluster To Array(cluster=w794) -> (array=w793:i16[])
        n426 = To Unsigned Long Integer(number=w793) -> (unsigned 32bit integer=w774:u32[])
        n427 = local read "Scan steps (AOD)"() -> (w795:u64)
        n428 = Multiply(x=w785, y="N Acq Sets (Traps + Fl.)") -> (x*y=w783:u32)
        n429 = Divide(x=40000000.0, y=w785) -> (x/y=w777:dbl)
        "AI rate (Hz)" <- w777
        "Ave. Rate (Hz)" <- w777
        n430 = Add Array Elements(numeric array=w774) -> (sum=w786:u32)
        "Trap Sets" <- w786
        n431 = Reciprocal(x=w777) -> (1/x=→"Ave. Period (s)":dbl)
        n432 = property on="Scan steps (AOD)" class="DigNum (strict)"("Val(Sgnl)"=w795) -> ()  [unwired: 2 in, 2 out]
        n433 = Divide(x=w777, y="N Acq Sets (Traps + Fl.)") -> (x/y=w799:dbl)
        "Data Rate (Hz)" <- w799
        n434 = Reciprocal(x=w799) -> (1/x=→"Data Period (s)":dbl)
        n435 = local read "Save ave N"() -> (w798:dbl)
        n436 = Divide(x=w799, y=w798) -> (x/y=w797:dbl)
        "Save Data Rate (Hz)" <- w797
        n437 = Reciprocal(x=w797) -> (1/x=→"Save Data Period (s)":dbl)
        n438 = Multiply(x=w783, y="# Samples/trap") -> (x*y=w781:u32)
        "Counts/DMA" <- w781
        n439 = property on="Trap Disp. Downsample" class="DigNum (strict)"("Maximum"="# Samples/trap") -> ()  [unwired: 2 in, 2 out]
        n440 = Multiply(x=w786, y="# Samples/trap") -> (x*y=w775:u32)
        "# Samples/channel" <- w775
        n441 = Multiply(x=w775, y=u32 8) -> (x*y=→"Trap AI Elements/DMA read":u32)
        n442 = local read "APD Int. Count"() -> (w782:u32)
        n443 = Multiply(x=w775, y=u32 3) -> (x*y=→"Trap Pos Elements/DMA read":u32)
        n444 = Divide(x=w781, y=w782) -> (x/y=w772:dbl)
        "APD Samples/FIFO Acq." <- w772
        n445 = Divide(x=w781, y=40000000.0) -> (x/y=w779:dbl)
        "DMA Update Period (s)" <- w779
        n446 = Multiply(x=2.0, y=w772) -> (x*y=→"APD Elements/DMA read":dbl)
        n447 = property on="APD Disp. Downsample" class="DigNum (strict)"("Maximum"=w772) -> ()  [unwired: 2 in, 2 out]
        n448 = local read "N sets to save"() -> (w791:u32)
        n449 = Multiply(x=w779, y=w791) -> (x*y=→"Total Time (s)":dbl)
        "FPGA Averaging" <- FALSE ("FPGA Averaging")
      }
      event "Rescale on Mean": Value Change {
        n450 = event-data() -> ()  [unwired: 7 out]
        n451 = And(x=FALSE, y="Rescale on Mean") -> (x .and. y?=w806:bool)
        n452 = local write "Rescale on Mean"(w806) -> ()
        n453 = local read "Bead Mean (nm)"() -> (w811:dbl)
        n454 = Add(x="Amplitude (nm)", y=w811) -> (x+y=w809:dbl)
        n455 = Subtract(x=w811, y="Amplitude (nm)") -> (x-y=w808:dbl)
        n456 = property on="Bead Separation" class="WFChart (strict)"("YScale.Minimum"=w808) -> ()  [unwired: 2 in, 2 out]
        n457 = property on="Bead Separation" class="WFChart (strict)"("YScale.Maximum"=w809) -> ()  [unwired: 2 in, 2 out]
      }
      event "Detector Type": Value Change {
        n458 = event-data() -> ()  [unwired: 7 out]
        n459 = local read "AI labels"() -> (w812:string[])
        n460 = property on="High Res. Display" class="Ring (strict)"("Strings []"=w812) -> ()  [unwired: 2 in, 2 out]
        n461 = Build Array (concatenate)(w812, "none") -> (w813:string[])
        n462 = property on="FFT 1 Choice 1" class="Ring (strict)"("Strings []"=w813) -> ()  [unwired: 2 in, 2 out]
        n463 = property on="FFT 1 Choice 2" class="Ring (strict)"("Strings []"=w813) -> ()  [unwired: 2 in, 2 out]
        n464 = property on="FFT 2 Choice 1" class="Ring (strict)"("Strings []"=w813) -> ()  [unwired: 2 in, 2 out]
        n465 = property on="FFT 2 Choice 2" class="Ring (strict)"("Strings []"=w813) -> ()  [unwired: 2 in, 2 out]
        n466 = Bundle("APD 1", "APD 2") -> (w816:cluster{string, string})  [unwired: 1 out]
        n467 = Cluster To Array(cluster=w816) -> (array=w814:string[])
        n468 = Build Array (concatenate)(w814, w813) -> (w818:string[])
        n469 = Array Size(array=w818) -> (size(s)=w819:i32)
        n470 = property on="Signals to Plot" class="LstBox (strict)"("Item Names"=w818) -> ()  [unwired: 2 in, 2 out]
        n471 = property on="Signals to Plot" class="LstBox (strict)"("Number of Rows"=w819) -> ()  [unwired: 2 in, 2 out]
        n472 = property on="All Signals" class="WFChart (strict)"("LegNumRows"=w819) -> ()  [unwired: 2 in, 2 out]
      }
      event "Adjust Scale\nto Mean": Value Change {
        n473 = event-data() -> ()  [unwired: 7 out]
        n474 = local read "APD 1 Rate (Hz)"() -> (w828:dbl)
        n475 = Multiply(x=1000.0, y="Above (kHz)") -> (x*y=w826:dbl)
        n476 = Multiply(x=1000.0, y="Below (kHz)") -> (x*y=w824:dbl)
        n477 = Add(x=w826, y=w828) -> (x+y=w821:dbl)
        n478 = Subtract(x=w828, y=w824) -> (x-y=w822:dbl)
        n479 = property on="APD Chart" class="WFChart (strict)"("YScale.Minimum"=w822) -> ()  [unwired: 2 in, 2 out]
        n480 = property on="APD Chart" class="WFChart (strict)"("YScale.Maximum"=w821) -> ()  [unwired: 2 in, 2 out]
      }
      event "Phase adj. (AI1)", "+ phase (AI1)", "- phase (AI1)": Value Change {
        n481 = event-data() -> ()  [unwired: 7 out]
        n482 = Negate(x="Phase adj. (AI1)") -> (-x=w838:i16)
        n483 = Select(t=w838, s="- phase (AI1)", f="Phase adj. (AI1)") -> (s? t:f=w837:i16)
        n484 = xnode "Read/Write Control"("FPGA VI Reference In"=w841, "error in"=w840, "Phase count adjustment"=w837) -> ("FPGA VI Reference Out"=w836:T20, "error out"=w835:errorcluster)
        n485 = Or(x="- phase (AI1)", y="+ phase (AI1)") -> (x .or. y?=w832:bool)
